vi "DLETETest Upload to S3.vi"() -> ()   [LabVIEW 2019]
uses:
  Control Experiment/Control Experiment.lvclass/Control Experiment.ctl
  Control Experiment/Control Experiment.lvclass
panel:
  in  "file to upload":path
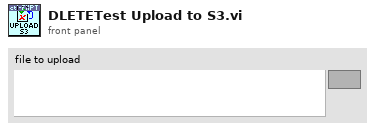
[diagram p1: front panel]
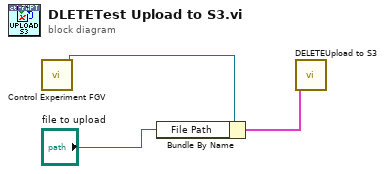
[diagram p0: block diagram]
diagram:
  n1 = call "Control Experiment FGV.vi"() -> ("Control Experiment.lvclass out"=w3:refnum<class "Control Experiment.lvclass">)  [unwired: 10 in, 1 out]
  n2 = Bundle By Name(cluster=w3, "File Path"="file to upload") -> (w1:cluster{})
  n3 = call "DELETEUpload to S3.vi"("Control Experiment in"=w1) -> ()  [unwired: 9 in, 2 out]
